vi "Configure Motor (Pulse Torque).vi"(0 "VISA resource name":refnum<visa-resource-name>, 2 "Scaling Factor (1.0000)":dbl=1.0 min=0.0001 max=99999.9999 format="%.4f", 5 "Pulse Range Upper (50.0000 N.m)":dbl=50.0 min=-10000.0 max=10000.0 format="%.4f", 7 "Pulse Range Lower (-50.0000 N.m)":dbl=-50.0 min=-10000.0 max=10000.0 format="%.4f", 9 "Rated Upper (50.0000 N.m)":dbl=50.0 min=-10000.0 max=10000.0 format="%.4f", 11 "error in (no error)":errorcluster, 12 "Rated Frequency Upper (15000 Hz)":i32=15000 min=1 max=100000000 step=1, 13 "Rated Lower (-50.0000 N.m)":dbl=-50.0 min=-10000.0 max=10000.0 format="%.4f", 14 "Rated Frequency Lower (5000 Hz)":i32=5000 min=1 max=100000000) -> (4 "VISA resource name out":refnum<visa-resource-name>, 15 "error out":errorcluster)   [LabVIEW 2021, in "Yokogawa WT1800 Series.lvlib"]
doc: "Configures the pulse torque motor features.\n\n<b>Note:</b>\nThis setting valid on models with the motor evaluation function (/MTR) option."
uses:
  <instrlib>/Yokogawa WT1800 Series/Yokogawa WT1800 Series.lvlib
panel:
  # "N.m"
  # "N.m"
  # "N.m"
  # "Hz"
  # "N.m"
  # "Hz"
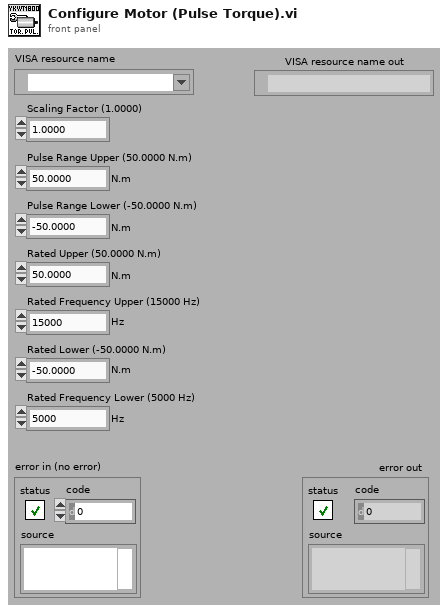
[diagram p1: front panel]
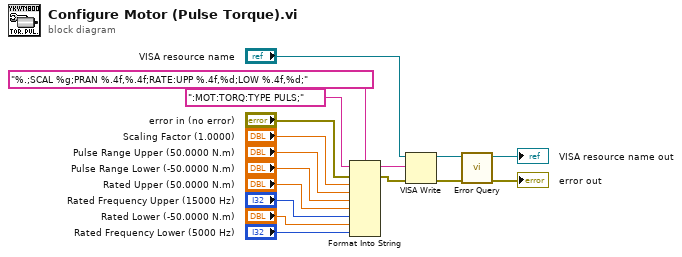
[diagram p0: block diagram]
diagram:
  n1 = Format Into String(format string="%.;SCAL %g;PRAN %.4f,%.4f;RATE:UPP %.4f,%d;LOW %.4f,%d;" ("形式文字列"), initial string=":MOT:TORQ:TYPE PULS;" ("形式文字列"), error in="error in (no error)", "Scaling Factor (1.0000)", "Pulse Range Upper (50.0000 N.m)", "Pulse Range Lower (-50.0000 N.m)", "Rated Upper (50.0000 N.m)", "Rated Frequency Upper (15000 Hz)", "Rated Lower (-50.0000 N.m)", "Rated Frequency Lower (5000 Hz)") -> (resulting string=w6:string, error out=w5:errorcluster)
  n2 = VISA Write ("VISA書き込み")(VISA resource name="VISA resource name", write buffer=w6, error in (no error)=w5) -> (VISA resource name out=w17:refnum<visa-resource-name>, error out=w16:errorcluster)  [unwired: 1 out]
  n3 = call <instrlib>:"Error Query.vi"("error in (no error)"=w16, "VISA resource name"=w17) -> ("error out"=→"error out":errorcluster, "VISA resource name out"=→"VISA resource name out":refnum<visa-resource-name>)  [unwired: 6 in, 2 out]
